vi "Close Communications.vi"(8 "error in (no error)":errorcluster, 10 "Final Stop?":bool, 11 "SCADA Communications in":refnum<class "SCADA Communications.lvclass">) -> (0 "error out":errorcluster, 3 "SCADA Communications out":refnum<class "SCADA Communications.lvclass">)   [LabVIEW 2015, in "SCADA Communcations Actor.lvlib" / "SCADA Communications.lvclass"]
uses:
  SCADA Communications.lvclass
  <vilib>/ActorFramework/Actor/Actor.lvclass/Actor.ctl
  <vilib>/ActorFramework/Message Enqueuer/Message Enqueuer.lvclass/Message Enqueuer.ctl
  <vilib>/ActorFramework/Message Enqueuer/Enqueue.vi
  <vilib>/ActorFramework/Message Priority Queue/Priority Enqueue.vi
  TCPIP Communications Framework/TCPIP Communications/TCPIP Communications.lvclass
  Master Controller Core/Master Controller Messages/Restart SCADA Msg/Restart SCADA Msg.lvclass
  <vilib>/ActorFramework/Actor/Actor.lvclass
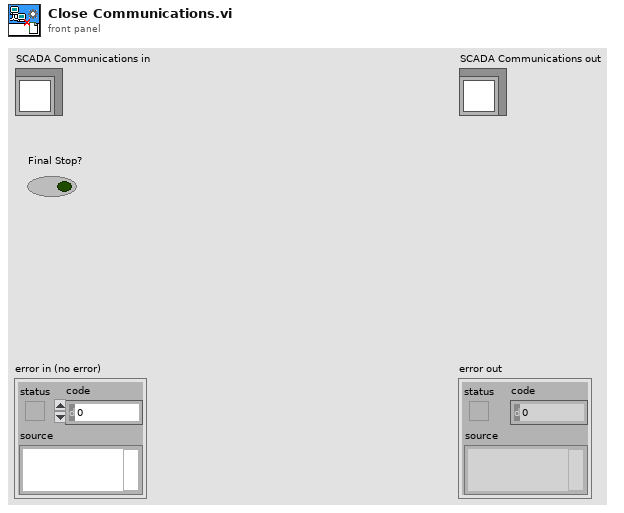
[diagram p1: front panel]
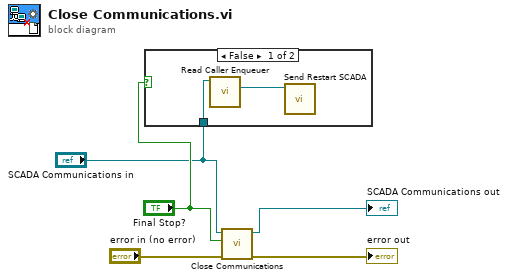
[diagram p0: block diagram]
diagram:
  n1 = case shown="False" "Final Stop?" {
    tunnel: "SCADA Communications in" -> [w7 _]
    frame False {
      n2 = call <vilib>:"Read Caller Enqueuer.vi"("Actor"=w7) -> ("Caller Enqueuer"=w6:refnum<class "Message Enqueuer.lvclass">)  [unwired: 10 in]
      n3 = call "Send Restart SCADA.vi"("Message Enqueuer"=w6) -> ()  [unwired: 9 in, 2 out]
    }
    frame True {
    }
  }
  n4 = call-parent "Close Communications.vi"("error in (no error)"="error in (no error)", "Final Stop?"="Final Stop?", "TCPIP Communications in"="SCADA Communications in") -> ("error out"=→"error out":errorcluster, "TCPIP Communications out"=→"SCADA Communications out":refnum<class "SCADA Communications.lvclass">)  [unwired: 7 in]
